vi "getDataFromTDMS.vi"(11 "文件名称":string="test") -> (3 "数据":string[][](array[string]))   [LabVIEW 2017]
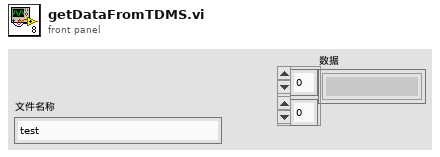
[diagram p1: front panel]
types:
  T1 = enum16{"open", "open or create", "create or replace", "create", "open (read-only)"}
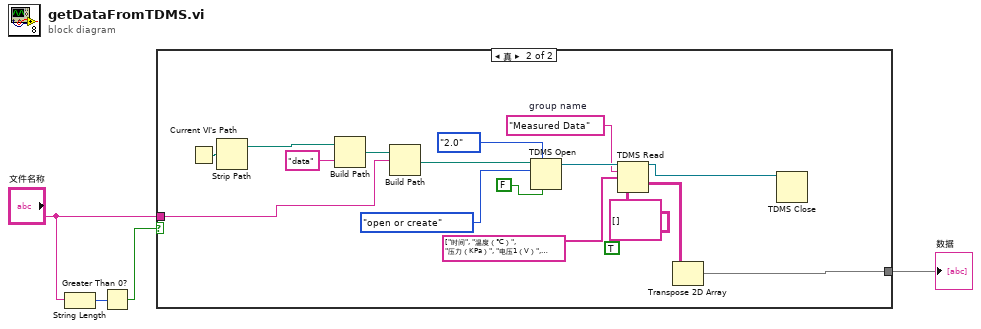
[diagram p0: block diagram]
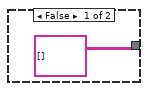
[diagram p2: hidden frame]
diagram:
  n1 = String Length(string="文件名称") -> (length=w2:i32)
  n2 = Greater Than 0?(x=w2) -> (x > 0?=w1:bool)
  n3 = case shown="真" w1 {
    tunnel: [string[][] [] w9] -> w4
    tunnel: "文件名称" -> [_ w7]
    frame False {
    }
    frame True {
      (unwired) TRUE ("文件结束？")
      w13 = "Measured Data"  # group name
      n4 = Current VI's Path() -> (path=w20:path)
      n5 = Strip Path(path=w20) -> (stripped path=w19:path)  [unwired: 1 out]
      n6 = Build Path(base path=w19, name or relative path="data" ("字符串")) -> (appended path=w8:path)
      n7 = Build Path(base path=w8, name or relative path=w7) -> (appended path=w21:path)
      n8 = TDMS Open(6:FALSE ("disable buffering (T)"), 7:enum16{"1.0", "2.0"}."2.0" ("file format version (2.0)"), 10:T1."open or create" ("operation"), 11:w21) -> (3:w14:refnum<k34>)  [unwired: 3 in, 1 out]
      n9 = TDMS Read(0:w14, 5:w13, 7:string[] ["时间", "温度（℃）", "压力（KPa）", "电压1（V）", "桥压1（V）", "电压2（V）", "桥压2（V）", "电压3（V）", "桥压3（V）", "电压4（V）", "桥压4（V）", "电压5（V）", "桥压5（V）", "电压6（V）", "桥压6（V）", "电压7（V)", "桥压7（V)", "电压8（V）", "桥压8（V）", "电压9（V)", "桥压9（V）", "电压10（V)", "桥压10（V）"], 12:string[][] []) -> (4:w11:refnum<k34>, 10:w10:string[][])  [unwired: 4 in, 4 out]
      n10 = Transpose 2D Array(2D array=w10) -> (transposed array=w9:string[][])
      n11 = TDMS Close(11:w11) -> ()  [unwired: 1 in, 2 out]
    }
  }
  "数据" <- w4
